vi "POLARIS Camera.vi"() -> ()   [LabVIEW 2014]
doc: "This VI is the default camera programm using IMAQdx Cam class and POLARIS Vision Display.\n\nIf runs als EXE please provide COMMAND LINE PARAMETERS: \n--\"Cameraname\" \"Config Dir\" \"FP Title\" \"Work Dir\" \n\nauthor: Alexander Kessler, Helmholtz-Institut-Jena \nmaintainer: Alexander Kessler: alexander.kessler@uni-jena.de\n\n\n\nLicense Agreement for this software:\n\nCopyright (C)\nHelmholtz-Institut-Jena\nFröbelstieg 3\n07743 Jena\nGermany\n\nThis program is free software; you can redistribute it and/or modify it under the terms of the GNU General Public License as published by the Free Software Foundation; either version 2 of the license, or (at your option) any later version.\n\nThis program is distributed in the hope that it will be useful, but WITHOUT ANY WARRANTY; without even the implied warranty of MERCHANTABILITY or FITNESS FOR A PARTICULAR PURPOSE. See the GNU General License for more details (http://www.gnu.org)."
uses:
  XDisplay/POLARIS IMAQ Display.xctl
  <vilib>/userdefined/High Color/IMAQdx.ctl
  IMAQdx Cam/IMAQdx Cam.lvclass
  XDisplay/Properties/ImageSource.ctl
  Analyze Classes/Analyze Diviation/Analyze BeamDeviation.lvclass
panel:
  in  "Settings":enum32{"Page 1"}(tab)
  in  "WorkDir":path=path "D:/Test XDisplay images"
  in  "Config Dir":path=path "D:/Test XDisplay images"
  in  "OK Button":bool
  out "XDisplay":cluster{"Image":T1}(xcontrol)
  in  "Camera":T2
  in  "Show settings":bool
  in  "stop2":bool
  in  "Prefix":string
  in  "stop":bool
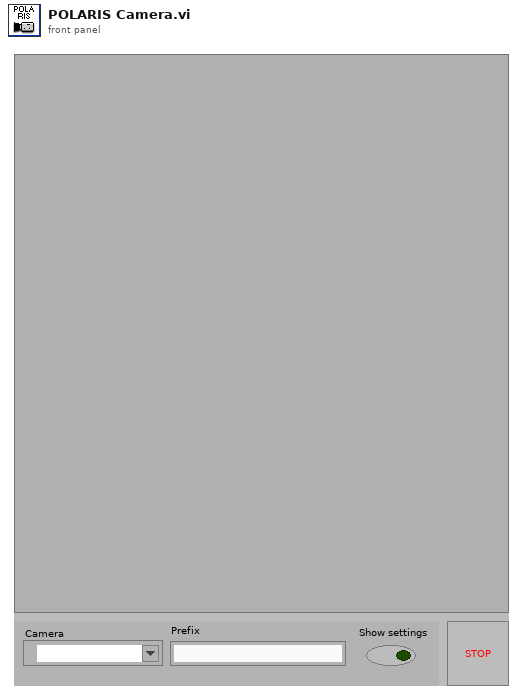
[diagram p1: front panel]
types:
  T1 = typedef "IMAQ Image.ctl" = refnum<image>
  T2 = typedef "IMAQdx.ctl" = refnum<k21>
  T3 = typedef "POLARIS IMAQ Display.xctl/ImageSource.ctl" = enum16{"Camera", "File"}
  T4 = typedef "Image Type" = u32
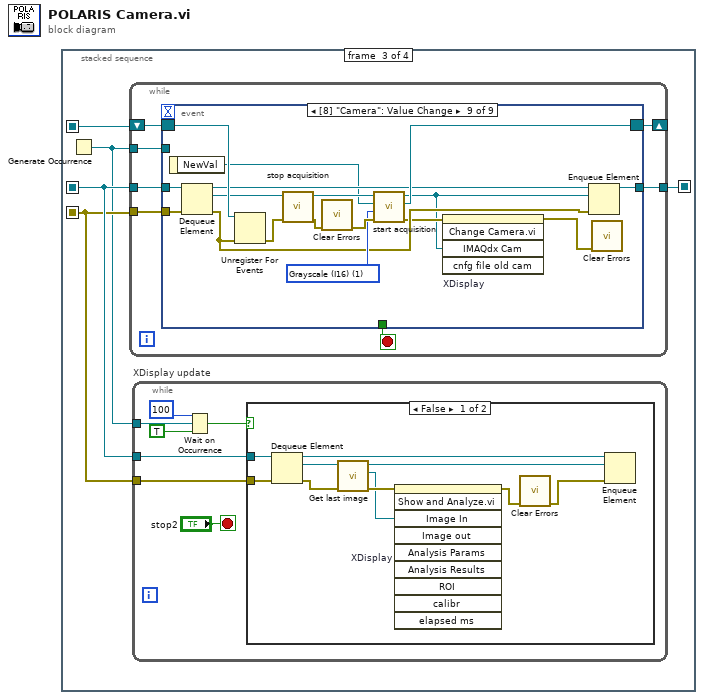
[diagram p0: block diagram]
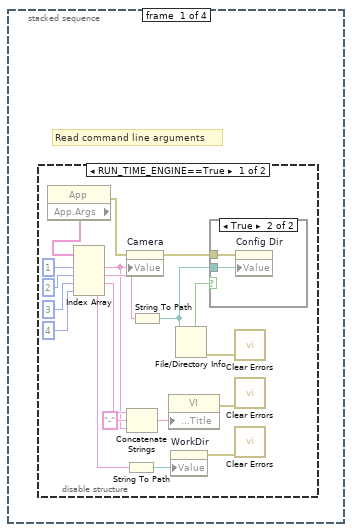
[diagram p2: hidden frame]
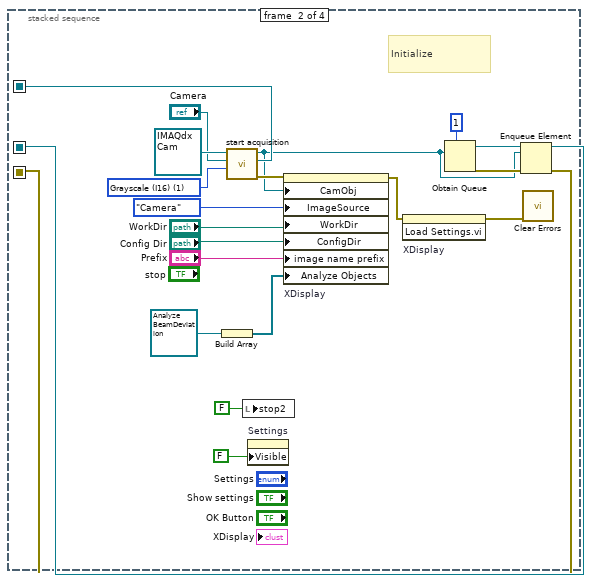
[diagram p5: hidden frame]
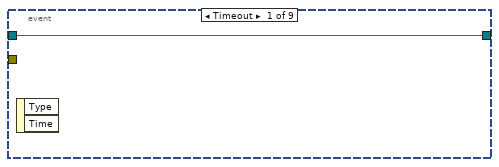
[diagram p7: hidden frame]
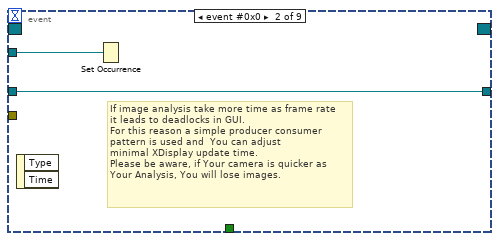
[diagram p8: hidden frame]
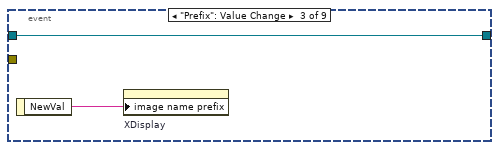
[diagram p9: hidden frame]
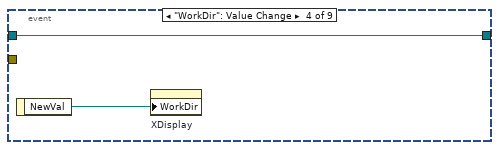
[diagram p10: hidden frame]
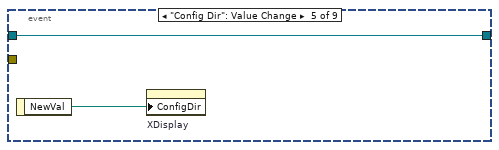
[diagram p11: hidden frame]
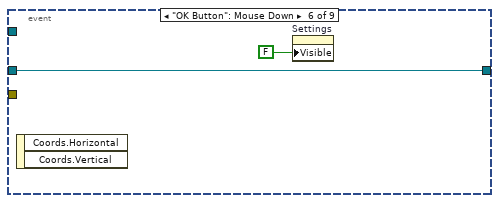
[diagram p12: hidden frame]
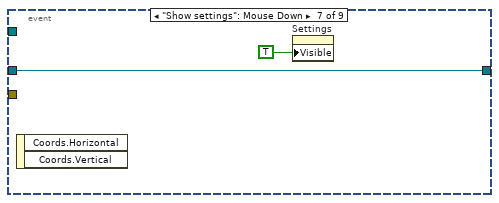
[diagram p13: hidden frame]
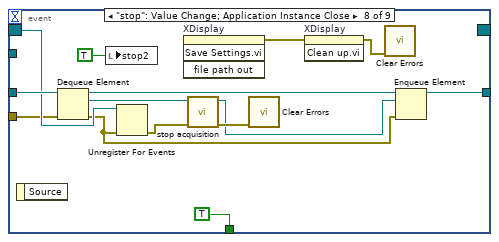
[diagram p14: hidden frame]
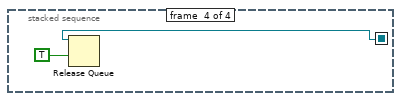
[diagram p15: hidden frame]
diagram:
  n1 = stacked-sequence {
    seq-local: [_ w42 _ _] -> [_ _ w47 _]
    seq-local: [_ w29 _ _] -> [_ _ w46 _]
    seq-local: [_ w28 _ _] -> [_ _ w45 _]
    seq-local: [_ _ w44 _] -> [_ _ _ w117]
    frame #0 {
      # "Read command line arguments"
      n2 = disable-structure shown="RUN_TIME_ENGINE==True" {
        frame condition #0 {
          n3 = property class="App"() -> (error out=w13:errorcluster, "App.Args"=w19:string[])  [unwired: 2 in, 1 out]
          n4 = Index Array(array=w19, index #1=1 ("index"), index #2=2 ("index"), index #3=3 ("index"), index #4=4 ("index")) -> (element #1=w6:string, element #2=w18:string, element #3=w8:string, element #4=w4:string)
          n5 = String To Path(string=w4) -> (path=w3:path)
          n6 = property on="Camera" class="IMAQdx (strict)"(error in=w13, "Value"=w6) -> (error out=w17:errorcluster)  [unwired: 1 in, 1 out]
          n7 = Concatenate Strings(w8, "-" ("string"), w6) -> (w5:string)
          n8 = String To Path(string=w18) -> (path=w16:path)
          n9 = property class="VI"("Front Panel.Title"=w5) -> (error out=w1:errorcluster)  [unwired: 2 in, 1 out]
          n10 = property on="WorkDir" class="Path"("Value"=w3) -> (error out=w2:errorcluster)  [unwired: 2 in, 1 out]
          n11 = File/Directory Info(path=w16) -> (directory=w15:bool, error out=w14:errorcluster)  [unwired: 1 in, 5 out]
          n12 = case shown="True" w15 {
            tunnel: w16 -> [_ w21]
            tunnel: w17 -> [_ w20]
            frame False {
            }
            frame True {
              n13 = property on="Config Dir" class="Path"(error in=w20, "Value"=w21) -> ()  [unwired: 1 in, 2 out]
            }
          }
          n14 = call <vilib>:"Clear Errors.vi"("error in (no error)"=w14) -> ()  [unwired: 5 in, 2 out]
          n15 = call <vilib>:"Clear Errors.vi"("error in (no error)"=w1) -> ()  [unwired: 5 in, 2 out]
          n16 = call <vilib>:"Clear Errors.vi"("error in (no error)"=w2) -> ()  [unwired: 5 in, 2 out]
        }
        frame condition #1 (active) {
        }
      }
    }
    frame #1 {
      w37 = T4 1 items=["Grayscale (U8)", "Grayscale (I16)", "Grayscale (SGL)", "Complex (CSG)", "RGB (U32)", "HSL (U32)", "RGB (U64)", "Grayscale (U16)"] ("Image Type")
      # "Initialize"
      n17 = Build Array(refnum<class "Analyze BeamDeviation.lvclass"> refnum ("Analyze.lvlib:Analyze BeamDeviation.lvclass")) -> (w24:refnum<class "Analyze BeamDeviation.lvclass">[])
      n18 = call-dynamic "start acquisition.vi"("Image Type"=w37, "Camera Name"="Camera", "IMAQdx Cam in"=refnum<class "IMAQdx Cam.lvclass"> refnum ("IMAQdx Cam.lvclass")) -> ("error out"=w38:errorcluster, "Event Registration Refnum"=w42:refnum<event-registration>, "IMAQdx Cam out"=w30:refnum<class "IMAQdx Cam.lvclass">)  [unwired: 6 in]
      n19 = local write "stop2"(FALSE ("stop2")) -> ()
      n20 = property on="Settings" class="TabCtl (strict)"("Visible"=FALSE) -> ()  [unwired: 2 in, 2 out]
      n21 = property on="XDisplay" class="POLARIS IMAQ Display (strict)"(error in=w38, "CamObj"=w30, "ImageSource"=ImageSource."Camera", "WorkDir"="WorkDir", "ConfigDir"="Config Dir", "image name prefix"="Prefix", "Analyze Objects"=w24) -> (error out=w26:errorcluster)  [unwired: 1 in, 1 out]
      n22 = invoke on="XDisplay" class="POLARIS IMAQ Display (strict)" method="Load Settings.vi"(error in=w26) -> (error out=w25:errorcluster)  [unwired: 2 in, 2 out]
      n23 = Obtain Queue(max queue size (-1, unlimited)=1, element data type=w30) -> (queue out=w32:refnum<queue>, error out=w31:errorcluster)  [unwired: 3 in, 1 out]
      n24 = Enqueue Element(queue=w32, element=w30, error in (no error)=w31) -> (queue out=w29:refnum<queue>, error out=w28:errorcluster)  [unwired: 1 in, 1 out]
      n25 = call <vilib>:"Clear Errors.vi"("error in (no error)"=w25) -> ()  [unwired: 5 in, 2 out]
    }
    frame #2 {
      n26 = Generate Occurrence() -> (w43:refnum<k4>)
      n27 = while {
        tunnel: w43 -> [w68]
        shift-right: [w67] -> _
        shift-left: w47 -> [w69]
        tunnel: w45 -> [w66]
        tunnel: w46 -> [w70]
        tunnel: [w65] -> w44
        stop <- w71 stop-if-true
        n28 = event shown="[8] \"Camera\": Value Change" {
          selector: w69 -> [_ _ _ _ _ _ _ w95 w110]
          dyn-events: [_ _ _ _ _ _ _ _ w111] -> w67
          timeout: _ -> [_ _ _ _ _ _ _ _ _]
          tunnel: [_ _ _ _ _ _ _ TRUE _] -> w71
          tunnel: w70 -> [w72 w73 w75 w77 w79 w81 w83 w96 w108]
          tunnel: w68 -> [_ w74 _ _ _ _ _ _ _]
          tunnel: [w72 w73 w75 w77 w79 w81 w83 w89 w104] -> w65
          tunnel: w66 -> [_ _ _ _ _ _ _ w87 w106]
          event Timeout {
            n29 = event-data() -> ()  [unwired: 1 in, 2 out]
          }
          event event #0x0 {
            # "If image analysis take more time as frame rate\nit leads to deadlocks in GUI.\nFor this reason a simple producer consumer \npattern is used and  You can adjust \nminimal XDisplay update time.\nPlease be aware, if Your camera is quicker as\nYour Analysis, You will lose images."
            n30 = event-data() -> ()  [unwired: 1 in, 2 out]
            n31 = Set Occurrence(w74) -> ()
          }
          event "Prefix": Value Change {
            n32 = event-data() -> ("NewVal"=w76:string)  [unwired: 1 in]
            n33 = property on="XDisplay" class="POLARIS IMAQ Display (strict)"("image name prefix"=w76) -> ()  [unwired: 2 in, 2 out]
          }
          event "WorkDir": Value Change {
            n34 = event-data() -> ("NewVal"=w78:path)  [unwired: 1 in]
            n35 = property on="XDisplay" class="POLARIS IMAQ Display (strict)"("WorkDir"=w78) -> ()  [unwired: 2 in, 2 out]
          }
          event "Config Dir": Value Change {
            n36 = event-data() -> ("NewVal"=w80:path)  [unwired: 1 in]
            n37 = property on="XDisplay" class="POLARIS IMAQ Display (strict)"("ConfigDir"=w80) -> ()  [unwired: 2 in, 2 out]
          }
          event "OK Button": Mouse Down {
            n38 = event-data() -> ()  [unwired: 1 in, 2 out]
            n39 = property on="Settings" class="TabCtl (strict)"("Visible"=FALSE) -> ()  [unwired: 2 in, 2 out]
          }
          event "Show settings": Mouse Down {
            n40 = event-data() -> ()  [unwired: 1 in, 2 out]
            n41 = property on="Settings" class="TabCtl (strict)"("Visible"=TRUE) -> ()  [unwired: 2 in, 2 out]
          }
          event "stop": Value Change; Application Instance Close {
            n42 = event-data() -> ()  [unwired: 1 in, 1 out]
            n43 = Dequeue Element(queue=w96, error in (no error)=w87) -> (queue out=w90:refnum<queue>, element=w91:refnum<class "IMAQdx Cam.lvclass">, error out=w86:errorcluster)  [unwired: 1 in, 1 out]
            n44 = local write "stop2"(TRUE ("stop2")) -> ()
            n45 = Unregister For Events(event registration refnum=w95, error in=w86) -> (error out=w97:errorcluster)
            n46 = invoke on="XDisplay" class="POLARIS IMAQ Display (strict)" method="Save Settings.vi"() -> (error out=w92:errorcluster)  [unwired: 4 in, 3 out]
            n47 = call-dynamic "stop acquisition.vi"("error in (no error)"=w97, "IMAQdx Cam in"=w91) -> ("error out"=w94:errorcluster, "IMAQdx Cam out"=w88:refnum<class "IMAQdx Cam.lvclass">)  [unwired: 8 in]
            n48 = call <vilib>:"Clear Errors.vi"("error in (no error)"=w94) -> ()  [unwired: 5 in, 2 out]
            n49 = invoke on="XDisplay" class="POLARIS IMAQ Display (strict)" method="Clean up.vi"(error in=w92) -> (error out=w85:errorcluster)  [unwired: 2 in, 2 out]
            n50 = call <vilib>:"Clear Errors.vi"("error in (no error)"=w85) -> ()  [unwired: 5 in, 2 out]
            n51 = Enqueue Element(queue=w90, element=w88, error in (no error)=w86) -> (queue out=w89:refnum<queue>)  [unwired: 1 in, 2 out]
          }
          event Value Change {
            w112 = T4 1 items=["Grayscale (U8)", "Grayscale (I16)", "Grayscale (SGL)", "Complex (CSG)", "RGB (U32)", "HSL (U32)", "RGB (U64)", "Grayscale (U16)"] ("Image Type")
            n52 = event-data() -> ("NewVal"=w100:T2)  [unwired: 1 in]
            n53 = Dequeue Element(queue=w108, error in (no error)=w106) -> (queue out=w105:refnum<queue>, element=w107:refnum<class "IMAQdx Cam.lvclass">, error out=w102:errorcluster)  [unwired: 1 in, 1 out]
            n54 = Unregister For Events(event registration refnum=w110, error in=w102) -> (error out=w109:errorcluster)
            n55 = call-dynamic "stop acquisition.vi"("error in (no error)"=w109, "IMAQdx Cam in"=w107) -> ("error out"=w115:errorcluster, "IMAQdx Cam out"=w113:refnum<class "IMAQdx Cam.lvclass">)  [unwired: 8 in]
            n56 = call <vilib>:"Clear Errors.vi"("error in (no error)"=w115) -> ("error out"=w114:errorcluster)  [unwired: 5 in, 1 out]
            n57 = call-dynamic "start acquisition.vi"("error in (no error)"=w114, "Image Type"=w112, "Camera Name"=w100, "IMAQdx Cam in"=w113) -> ("error out"=w101:errorcluster, "Event Registration Refnum"=w111:refnum<event-registration>, "IMAQdx Cam out"=w99:refnum<class "IMAQdx Cam.lvclass">)  [unwired: 5 in]
            n58 = invoke on="XDisplay" class="POLARIS IMAQ Display (strict)" method="Change Camera.vi"(error in=w101, "IMAQdx Cam"=w99) -> (error out=w103:errorcluster)  [unwired: 3 in, 4 out]
            n59 = Enqueue Element(queue=w105, element=w99, error in (no error)=w102) -> (queue out=w104:refnum<queue>)  [unwired: 1 in, 2 out]
            n60 = call <vilib>:"Clear Errors.vi"("error in (no error)"=w103) -> ()  [unwired: 5 in, 2 out]
          }
        }
      }
      n61 = while "XDisplay update" {
        tunnel: w43 -> [w54]
        tunnel: w46 -> [w51]
        tunnel: w45 -> [w50]
        stop <- "stop2" stop-if-true
        n62 = Wait on Occurrence(1:TRUE ("ignore previous (T)"), 2:w54, 3:100 ("ms timeout (-1)")) -> (0:w52:bool)
        n63 = case shown="False" w52 {
          tunnel: w51 -> [w61 _]
          tunnel: w50 -> [w59 _]
          frame False {
            n64 = Dequeue Element(queue=w61, error in (no error)=w59) -> (queue out=w60:refnum<queue>, element=w57:refnum<class "IMAQdx Cam.lvclass">, error out=w58:errorcluster)  [unwired: 1 in, 1 out]
            n65 = call-dynamic "Get last image.vi"("error in (no error)"=w58, "IMAQdx Cam in"=w57) -> ("error out"=w64:errorcluster, "Image Out"=w63:T1, "IMAQdx Cam out"=w56:refnum<class "IMAQdx Cam.lvclass">)  [unwired: 6 in, 1 out]
            n66 = invoke on="XDisplay" class="POLARIS IMAQ Display (strict)" method="Show and Analyze.vi"(error in=w64, "Image In"=w63) -> (error out=w62:errorcluster)  [unwired: 8 in, 9 out]
            n67 = call <vilib>:"Clear Errors.vi"("error in (no error)"=w62) -> ("error out"=w55:errorcluster)  [unwired: 5 in, 1 out]
            n68 = Enqueue Element(queue=w60, element=w56, error in (no error)=w55) -> ()  [unwired: 1 in, 3 out]
          }
          frame True {
          }
        }
      }
    }
    frame #3 {
      n69 = Release Queue(queue=w117, force destroy? (F)=TRUE) -> ()  [unwired: 1 in, 3 out]
    }
  }
